vi "Save_interim_img_mcores.vi"() -> ()   [LabVIEW 2020]
uses:
  <vilib>/Utility/file.llb/Write Delimited Spreadsheet (I64).vi
panel:
  out "Elapsed time [ms]":u32
  in  "h":i32=10 min=1 max=5000 step=1
  in  "w":i32=1 min=1 max=5000 step=1
  out "error out":errorcluster
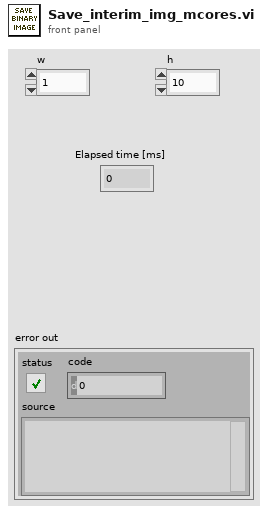
[diagram p1: front panel]
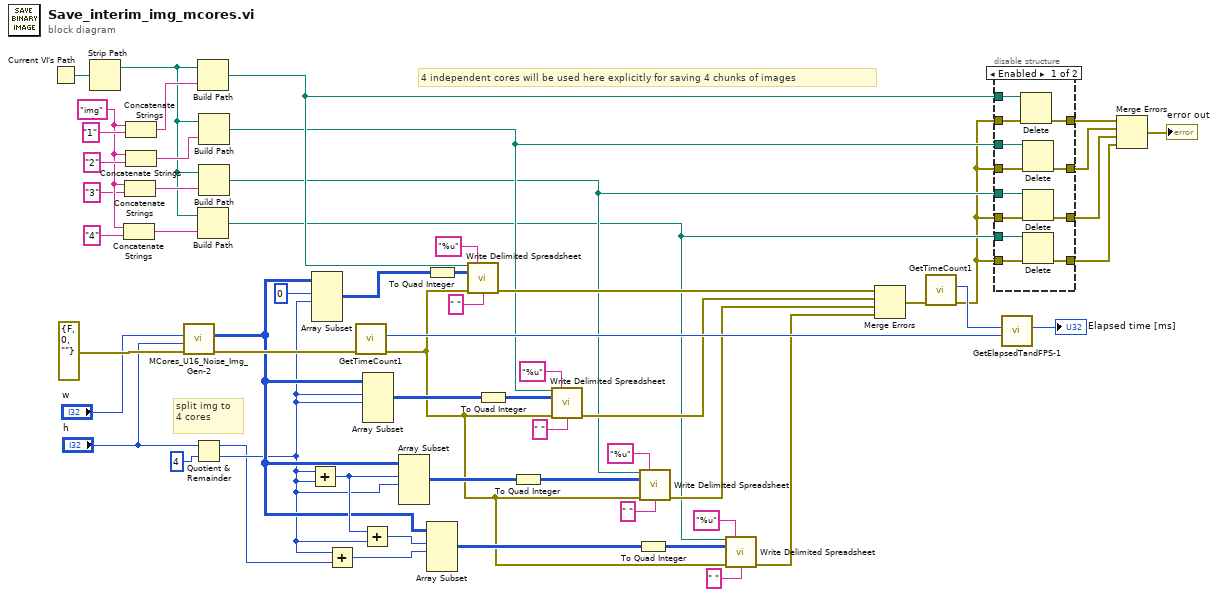
[diagram p0: block diagram]
diagram:
  w44 = "img" ("string")
  # "split img to\n4 cores"
  # "4 independent cores will be used here explicitly for saving 4 chunks of images"
  n1 = Current VI's Path() -> (path=w58:path)
  n2 = Strip Path(path=w58) -> (stripped path=w40:path)  [unwired: 1 out]
  n3 = Concatenate Strings(w44, "4" ("string")) -> (w39:string)
  n4 = Concatenate Strings(w44, "3" ("string")) -> (w41:string)
  n5 = Concatenate Strings(w44, "1" ("string")) -> (w47:string)
  n6 = Concatenate Strings(w44, "2" ("string")) -> (w45:string)
  n7 = call "MCores_U16_Noise_Img_Gen-2.vi"("error IN"=errorcluster {"status"=FALSE, "code"=0, "source"=""} ("error in (no error)"), "[IN] Width"="h", "[IN] Height"="w") -> ("error OUT"=w53:errorcluster, "[OUT] U16 Pixel Img"=w24:u16[][])  [unwired: 7 in]
  n8 = Quotient & Remainder(x="h", y=4) -> (x-y*floor(x/y)=w12:i32, floor(x/y)=w13:i32)
  n9 = Build Path(base path=w40, name or relative path=w47) -> (appended path=w10:path)
  n10 = Build Path(base path=w40, name or relative path=w39) -> (appended path=w7:path)
  n11 = Build Path(base path=w40, name or relative path=w45) -> (appended path=w9:path)
  n12 = Build Path(base path=w40, name or relative path=w41) -> (appended path=w8:path)
  n13 = Add(x=w13, y=w13) -> (x+y=w26:i32)
  n14 = Array Subset(array=w24, index (row)=0 ("index"), length (row)=w13) -> (w35:u16[][])  [unwired: 2 in]
  n15 = Add(x=w13, y=w12) -> (x+y=w11:i32)
  n16 = call "GetTimeCount1.vi"("error IN"=w53) -> ("error OUT"=w18:errorcluster, "[OUT] Timer Count"=w51:u32)  [unwired: 9 in]
  n17 = Add(x=w26, y=w13) -> (x+y=w25:i32)
  n18 = Array Subset(array=w24, index (row)=w13, length (row)=w13) -> (w31:u16[][])  [unwired: 2 in]
  n19 = Array Subset(array=w24, index (row)=w26, length (row)=w13) -> (w28:u16[][])  [unwired: 2 in]
  n20 = To Quad Integer(1:w35) -> (0:w55:i64[][])
  n21 = Array Subset(array=w24, index (row)=w25, length (row)=w11) -> (w20:u16[][])  [unwired: 2 in]
  n22 = call-poly <vilib>:"Write Delimited Spreadsheet.vi"("file path (dialog if empty)"=w10, "format (%d)"="%u", "2D data"=w55, "error in (no error)"=w18, "delimiter (\\t)"=" " ("delimiter (\\t)")) -> ("error out"=w21:errorcluster)  [unwired: 9 in, 1 out]
  n23 = To Quad Integer(1:w31) -> (0:w32:i64[][])
  n24 = To Quad Integer(1:w28) -> (0:w27:i64[][])
  n25 = call-poly <vilib>:"Write Delimited Spreadsheet.vi"("file path (dialog if empty)"=w9, "format (%d)"="%u", "2D data"=w32, "error in (no error)"=w18, "delimiter (\\t)"=" " ("delimiter (\\t)")) -> ("error out"=w16:errorcluster)  [unwired: 9 in, 1 out]
  n26 = To Quad Integer(1:w20) -> (0:w19:i64[][])
  n27 = call-poly <vilib>:"Write Delimited Spreadsheet.vi"("file path (dialog if empty)"=w8, "format (%d)"="%u", "2D data"=w27, "error in (no error)"=w18, "delimiter (\\t)"=" " ("delimiter (\\t)")) -> ("error out"=w15:errorcluster)  [unwired: 9 in, 1 out]
  n28 = call-poly <vilib>:"Write Delimited Spreadsheet.vi"("file path (dialog if empty)"=w7, "format (%d)"="%u", "2D data"=w19, "error in (no error)"=w18, "delimiter (\\t)"=" " ("delimiter (\\t)")) -> ("error out"=w14:errorcluster)  [unwired: 9 in, 1 out]
  n29 = Merge Errors(w21, w16, w15, w14) -> (w17:errorcluster)
  n30 = call "GetTimeCount1.vi"("error IN"=w17) -> ("error OUT"=w1:errorcluster, "[OUT] Timer Count"=w52:u32)  [unwired: 9 in]
  n31 = disable-structure shown="Enabled" {
    disable-tunnel: w10 -> [w70 _]
    disable-tunnel: w9 -> [w69 _]
    disable-tunnel: w8 -> [w68 _]
    disable-tunnel: w7 -> [w67 _]
    disable-tunnel: w1 -> [w66 w74]
    disable-tunnel: [w65 w74] -> w6
    disable-tunnel: [w64 w73] -> w5
    disable-tunnel: [w63 w72] -> w4
    disable-tunnel: [w62 w71] -> w3
    disable-tunnel: w1 -> [w61 w73]
    disable-tunnel: w1 -> [w60 w72]
    disable-tunnel: w1 -> [w59 w71]
    frame Enabled {
      n32 = Delete(path (use dialog)=w70, error in=w66) -> (error out=w65:errorcluster)  [unwired: 3 in, 2 out]
      n33 = Delete(path (use dialog)=w69, error in=w61) -> (error out=w64:errorcluster)  [unwired: 3 in, 2 out]
      n34 = Delete(path (use dialog)=w68, error in=w60) -> (error out=w63:errorcluster)  [unwired: 3 in, 2 out]
      n35 = Delete(path (use dialog)=w67, error in=w59) -> (error out=w62:errorcluster)  [unwired: 3 in, 2 out]
    }
    frame Disabled {
    }
  }
  n36 = call "GetElapsedTandFPS-1.vi"("[IN] Timer Count Before ALL [ms]"=w51, "[IN] Timer Count After ALL [ms]"=w52) -> ("[OUT] Elapsed time [ms]"=→"Elapsed time [ms]":u32)  [unwired: 3 in, 2 out]
  n37 = Merge Errors(w6, w5, w4, w3) -> (→"error out":errorcluster)
